vi "Get stack data_12042024.vi"(8 "error in (no error)":errorcluster, 11 "Stack in":refnum<class "Stack.lvclass">) -> (0 "error out":errorcluster, 2 "Data cluster":T1={"type"="proto", " geometry"="full", "resolution"="LD", "baselayer"="BA_123", "toplayer"="SI_789", "bl_pos"="1", "tl_pos"="1", "put_pos"="1", "region"="1", "asstray"="1", "comptray"="1", "put"="1", "date"="2024-04-02", "timestart"="1:12:12.442", "timeend"="1:23:45.244", "operator"="cmuperson", "tape"="some", "glue"="some", "stack name"="some", "Adhesive type"="", "Comments"="", "Temperature"="", "Relative Humidity"=""}, 3 "Stack out":refnum<class "Stack.lvclass">)   [LabVIEW 2021, in "Stack.lvclass"]
uses:
  Stack.lvclass
  Stack.lvclass/Stack.ctl
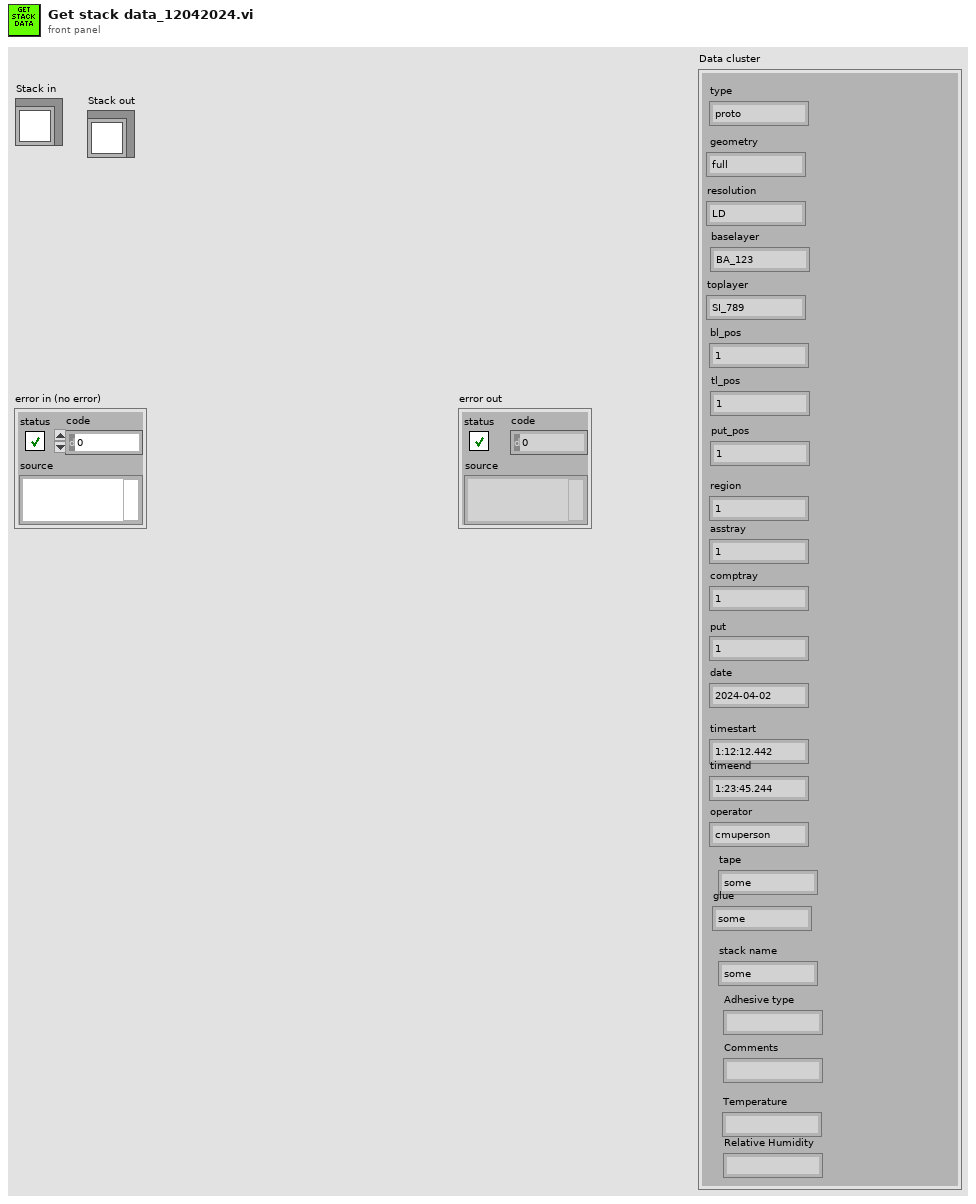
[diagram p1: front panel]
types:
  T1 = cluster{"type":string, " geometry":string, "resolution":string, "baselayer":string, "toplayer":string, "bl_pos":string, "tl_pos":string, "put_pos":string, "region":string, "asstray":string, "comptray":string, "put":string, "date":string, "timestart":string, "timeend":string, "operator":string, "tape":string, "glue":string, "stack name":string, "Adhesive type":string, "Comments":string, "Temperature":string, "Relative Humidity":string}
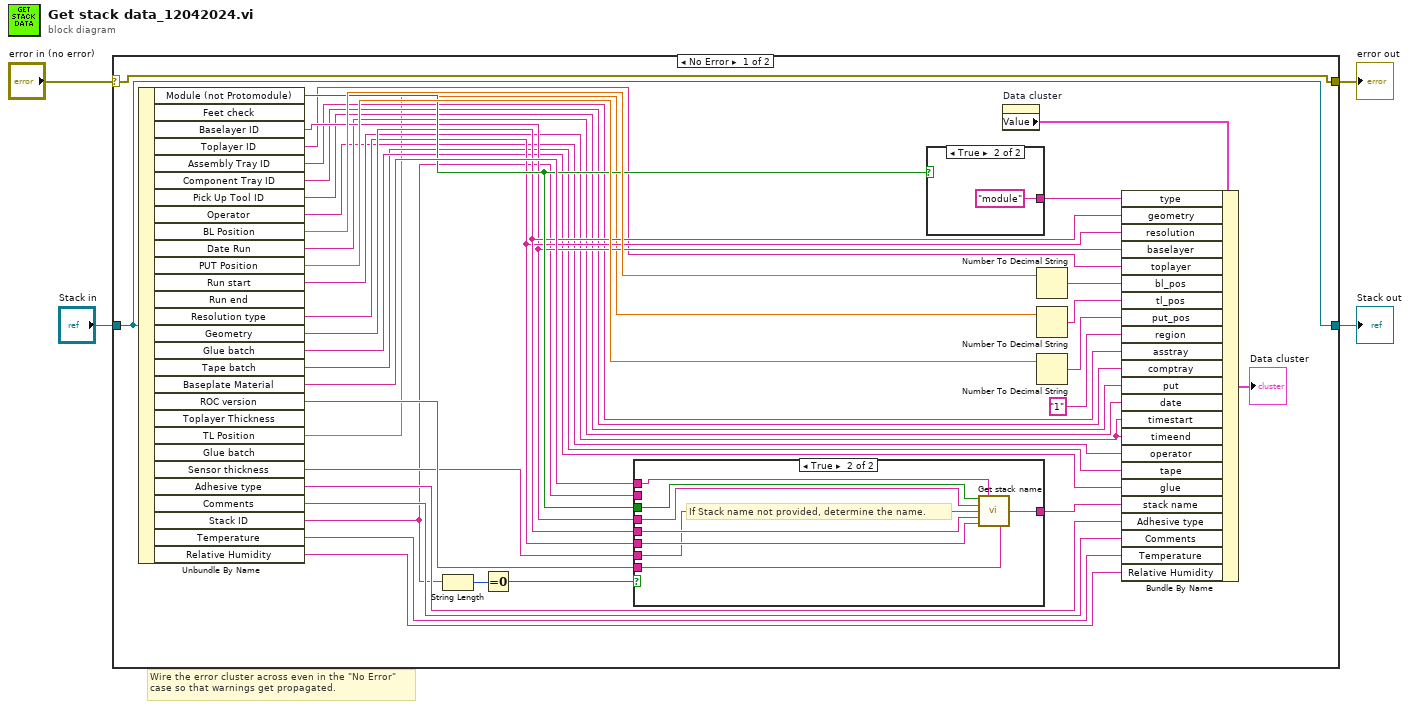
[diagram p0: block diagram]
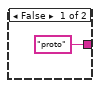
[diagram p3: hidden frame]
diagram:
  # "Wire the error cluster across even in the \"No Error\"\ncase so that warnings get propagated."
  n1 = case shown="No Error" "error in (no error)" {
    selector: "error in (no error)" -> [w40 w53]
    tunnel: [w40 w53] -> w3
    tunnel: [w39 w52] -> w1
    tunnel: "Stack in" -> [w39 w52]
    frame No Error {
      n2 = Unbundle By Name(w39) -> ("Module (not Protomodule)"=w35:bool, "Baselayer ID"=w27:string, "Toplayer ID"=w26:string, "Assembly Tray ID"=w25:string, "Component Tray ID"=w24:string, "Pick Up Tool ID"=w23:string, "Operator"=w20:string, "BL Position"=w38:dbl, "Date Run"=w22:string, "PUT Position"=w37:dbl, "Run start"=w21:string, "Resolution type"=w28:string, "Geometry"=w29:string, "Glue batch"=w19:string, "Tape batch"=w18:string, "Baseplate Material"=w36:string, "ROC version"=w34:string, "TL Position"=w17:dbl, "Sensor thickness"=w12:string, "Adhesive type"=w11:string, "Comments"=w10:string, "Stack ID"=w7:string, "Temperature"=w6:string, "Relative Humidity"=w5:string)  [unwired: 4 out]
      n3 = String Length(string=w7) -> (length=w9:i32)
      n4 = Equal To 0?(x=w9) -> (x = 0?=w8:bool)
      n5 = case shown="True" w8 {
        tunnel: w36 -> [_ w49]
        tunnel: w35 -> [_ w48]
        tunnel: w34 -> [_ w47]
        tunnel: [w41 w46] -> w31
        tunnel: w29 -> [_ w45]
        tunnel: w28 -> [_ w44]
        tunnel: w27 -> [_ w43]
        tunnel: w12 -> [_ w42]
        tunnel: w7 -> [w41 _]
        frame False {
        }
        frame True {
          # "If Stack name not provided, determine the name."
          n6 = call "Get stack name.vi"("Module?"=w48, "Baseplate Type"=w49, "Protoname (baselayer)"=w43, "Sensor thickness"=w42, "Geometry"=w45, "Resolution"=w44, "Hexaboard ROC version"=w47) -> ("Stack name"=w46:string)  [unwired: 8 in]
        }
      }
      n7 = case shown="True" w35 {
        tunnel: ["proto" ("type") "module" ("type")] -> w30
        frame False {
        }
        frame True {
        }
      }
      n8 = property on="Data cluster" class="Clust (strict)"() -> ("Value"=w32:T1)  [unwired: 2 in, 2 out]
      n9 = Number To Decimal String(number=w38) -> (decimal integer string=w15:string)  [unwired: 1 in]
      n10 = Number To Decimal String(number=w17) -> (decimal integer string=w16:string)  [unwired: 1 in]
      n11 = Number To Decimal String(number=w37) -> (decimal integer string=w14:string)  [unwired: 1 in]
      n12 = Bundle By Name(cluster=w32, "type"=w30, "geometry"=w29, "resolution"=w28, "baselayer"=w27, "toplayer"=w26, "bl_pos"=w15, "tl_pos"=w16, "put_pos"=w14, "region"="1", "asstray"=w25, "comptray"=w24, "put"=w23, "date"=w22, "timestart"=w21, "timeend"=w21, "operator"=w20, "tape"=w18, "glue"=w19, "stack name"=w31, "Adhesive type"=w11, "Comments"=w10, "Temperature"=w6, "Relative Humidity"=w5) -> (→"Data cluster":T1)
    }
    frame Error {
    }
  }
  "error out" <- w3
  "Stack out" <- w1
